vi "Read State from SHVs.vi"(8 "error in (no error)":errorcluster, 11 "Valve in":refnum<class "Valve.lvclass">) -> (0 "error out":errorcluster, 2 "BitField":u16, 3 "Valve out":refnum<class "Valve.lvclass">)   [LabVIEW 2015, in "cRIO-Carbondioxide.lvlib" / "CO2-Actor.lvlib" / "Valve.lvclass"]
uses:
  Valve.lvclass
  Valve.lvclass/Valve.ctl
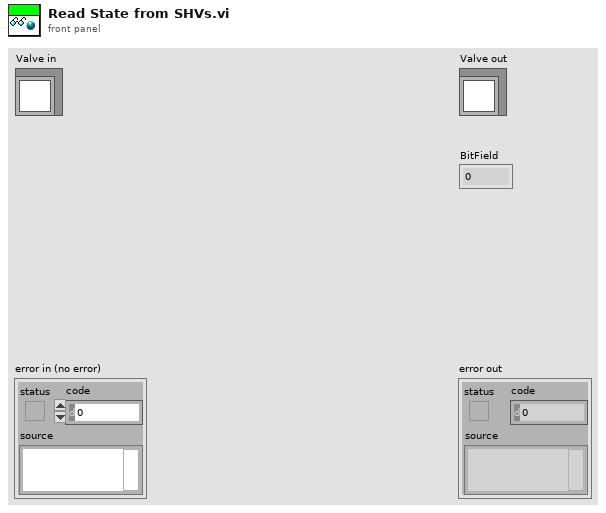
[diagram p1: front panel]
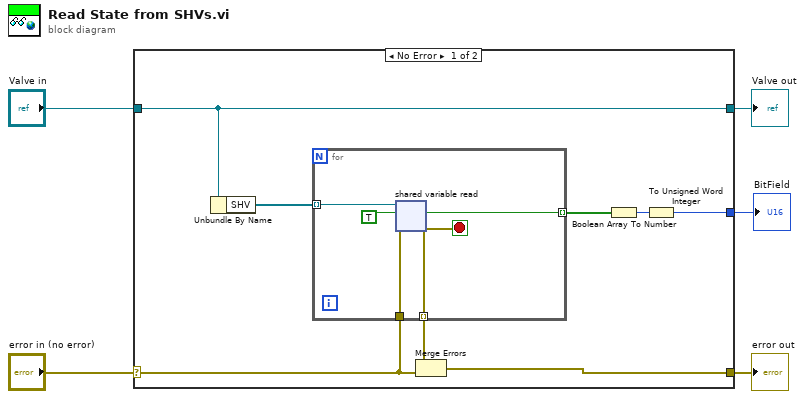
[diagram p0: block diagram]
diagram:
  n1 = case shown="No Error" "error in (no error)" {
    selector: "error in (no error)" -> [w11 w20]
    tunnel: [w10 w20] -> w4
    tunnel: [w13 w19] -> w2
    tunnel: "Valve in" -> [w13 w19]
    tunnel: [w6 _] -> w1
    frame No Error {
      n2 = Unbundle By Name(w13) -> ("SHV"=w12:refnum<k21>[])
      n3 = for {
        tunnel: w12 -> [w18] mode=indexing
        tunnel: w11 -> [w16]
        tunnel: [w15] -> w8 mode=indexing
        tunnel: [w14] -> w9 mode=indexing
        stop <- w14 stop-if-true
        n4 = shared-variable-read(w18, w16, TRUE) -> (w14:errorcluster, w15:bool)  [unwired: 2 out]
      }
      n5 = Merge Errors(w9, w11) -> (w10:errorcluster)
      n6 = Boolean Array To Number(Boolean array=w8) -> (number=w7:u32)
      n7 = To Unsigned Word Integer(number=w7) -> (unsigned 16bit integer=w6:u16)
    }
    frame Error {
    }
  }
  "error out" <- w4
  "Valve out" <- w2
  "BitField" <- w1
